vi "Caller.vi"(6 "Sub Panel":refnum<vi>, 8 "Error In":errorcluster, 10 "Data Value Reference In":refnum<data-value>, 11 "Divide In":refnum<class "Divide.lvclass">) -> (0 "Error Out":errorcluster, 3 "Divide Out":refnum<class "Divide.lvclass">)   [LabVIEW 2021, in "Calculator.lvlib" / "Divide.lvclass"]
doc: "This VI has controls and a boolean button in which user enters the input and the output is displayed when the calculate button is pressed. This VI is openend in the subpanel of main VI when the particular instance is choosen."
uses:
  Divide.lvclass
  UI.vi
  NumericOperation/NumericOperation.lvclass
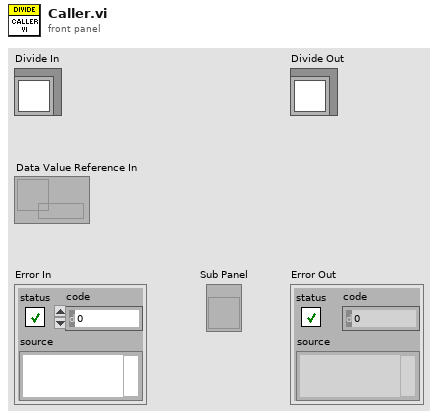
[diagram p1: front panel]
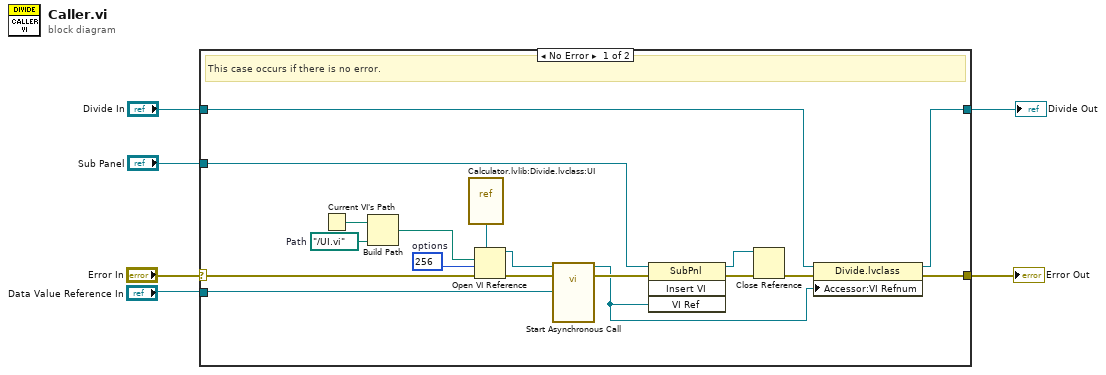
[diagram p0: block diagram]
diagram:
  n1 = case shown="No Error" "Error In" {
    selector: "Error In" -> [w24 w26]
    tunnel: [w13 w26] -> w5
    tunnel: [w10 w25] -> w3
    tunnel: "Divide In" -> [w12 w25]
    tunnel: "Sub Panel" -> [w15 _]
    tunnel: "Data Value Reference In" -> [w7 _]
    frame No Error {
      w14 = 256  # options
      w19 = path "../UI.vi"  # Path
      # "This case occurs if there is no error."
      n2 = Current VI's Path() -> (path=w20:path)
      n3 = Build Path(base path=w20, name or relative path=w19) -> (appended path=w21:path)
      n4 = vi-ref "Calculator.lvlib:Divide.lvclass:UI.vi"() -> (w18:refnum<vi>)
      n5 = Open VI Reference(type specifier VI Refnum (for type only)=w18, vi path=w21, options=w14, error in (no error)=w24) -> (vi reference=w17:refnum<vi>, error out=w23:errorcluster)  [unwired: 2 in]
      n6 = call-by-ref "Start Asynchronous Call"(reference=w17, error in=w23, "Data Value Reference In"=w7) -> (reference out=w11:refnum<vi>, error out=w22:errorcluster)  [unwired: 8 in, 3 out]
      n7 = invoke class="SubPnl" method="Insert VI"(reference=w15, error in=w22, "VI Ref"=w11) -> (reference out=w8:refnum<vi>, error out=w16:errorcluster)  [unwired: 1 in, 2 out]
      n8 = Close Reference(reference=w8, error in (no error)=w16) -> (error out=w9:errorcluster)
      n9 = property class="Divide.lvclass"(reference=w12, error in=w9, "Accessor:VI Refnum"=w11) -> (reference out=w10:refnum<class "Divide.lvclass">, error out=w13:errorcluster)
    }
    frame Error {
      # "This case occurs if there is any error"
    }
  }
  "Error Out" <- w5
  "Divide Out" <- w3
